vi "RT_Starting_Program.vi"() -> ()   [LabVIEW 2019]
uses:
  <vilib>/Simulation/Scripting/Companion Diagram/SimConfigNode/SimParams.ctl
  <vilib>/Simulation/Scripting/Companion Diagram/SimConfigNode/_simSolvers.ctl
  <vilib>/Simulation/Implementation/Shared/SIMSCR Execution Mode.ctl
  <vilib>/Platform/TimedLoop/XDataNode/timing_clust.ctl
  <vilib>/Platform/TimedLoop/XDataNode/nitl_modes.ctl
  <vilib>/Platform/TimedLoop/XDataNode/wakeup.ctl
  <vilib>/Simulation/Param Hierarchy/Typedefs/SIMPH Param Control Actions.ctl
  <vilib>/Simulation/Scripting/Editor Utilities/SIM subVI tag data.ctl
  <vilib>/Simulation/Scripting/Editor Utilities/SIM subVI execution type.ctl
  <vilib>/Simulation/Implementation/Shared/NILVSim_ParamChanged.vi
  <vilib>/Simulation/Implementation/Shared/NILVSim_FinishedLate.vi
  <vilib>/Simulation/Implementation/Shared/NILVSIM_BeginStep.vi
  <vilib>/Simulation/Utility/Implementation/SIM Halt.vi
  <vilib>/Simulation/Implementation/Shared/SIM Fire Discrete SubVI.vi
  <vilib>/Simulation/SignalDisplay/Implementation/NILVSim Time Waveform.llb/SIM Time Waveform (vector).vi
  <vilib>/Simulation/Implementation/Shared/NILVSim_Manager.vi
  <vilib>/Utility/error.llb/Clear Errors.vi
  <vilib>/Simulation/Implementation/Shared/NILVSim_FinalizeModel.vi
  <vilib>/Simulation/Implementation/Shared/SIM Fire Discrete SubVI (Core).vi
  <vilib>/myRIO/Common/Instrument Driver Framework/myRIO v1.0/UART/vis/myRIO v1.0 Close UART.vi
  <vilib>/FPGAPlugInAG/myRIO-1900/niLvFpga_Open_myRIO-1900.vi
  <vilib>/rvi/interface/common/dynamic/niFpgaDynamicAddResources.vi
  <vilib>/Utility/error.llb/Error Cluster From Error Code.vi
  <vilib>/rvi/errors/niLvFpgaAdjustHostInterfaceError.vi
  <vilib>/Simulation/Implementation/Shared/SIM Unbundle Sim Info.vi
  <vilib>/Simulation/Implementation/Shared/SIMSH Read Queue.vi
  <vilib>/Simulation/Implementation/Shared/NILVSim_Initialize.vi
  SubVIs/Output_Scaling.vi
  SubVIs/Encoder Scaling VI.vi
  <vilib>/Simulation/Utility/Implementation/NILVSim Get Time and IsAcceptedStep.vi
  <vilib>/Simulation/Implementation/Shared/NILVSim_GetModelError.vi
  <vilib>/Simulation/Implementation/Shared/SIM Bundle Sim Info.vi
  <vilib>/FPGAPlugInAG/Dynamic/niLvFpga_Close_Dynamic.vi
  <vilib>/myRIO/Common/Instrument Driver Framework/Utilities/vis/FPGA Ref Manager.vi
  <vilib>/myRIO/Common/Instrument Driver Framework/myRIO v1.0/myRIO v1.0 Reset FPGA.vi
  <vilib>/myRIO/Common/Instrument Driver Framework/myRIO v1.0/IRQ/vis/myRIO v1.0 IRQ Info FGV.vi
  <vilib>/myRIO/Common/Instrument Driver Framework/myRIO v1.0/IRQ/vis/myRIO v1.0 Timer IRQ Info FGV.vi
  <vilib>/myRIO/Common/Instrument Driver Framework/myRIO v1.0/IRQ/vis/myRIO v1.0 ISR Agent.vi
  <vilib>/myRIO/Instrument Drivers/Utilities/vis/Reset Index.vi
  <vilib>/myRIO/Common/Instrument Driver Framework/myRIO v1.0/Resource Manager/vis/myRIO v1.0 Block Write Resource Manager.vi
  <vilib>/rvi/interface/nirviOpenFPGA/nirviOpenFPGA.xnode
  FPGA Bitfiles/SheepdogProject_FPGATarget_FPGAEncoderandPW_gBORoPHN0GY.lvbitx
  <vilib>/rvi/interface/nirviReadWriteControl/nirviReadWriteControl.xnode
  <vilib>/Simulation/Scripting/Companion Diagram/SimConfigNode/SimDog.xnode
  <vilib>/Platform/TimedLoop/XDataNode/XDataNode.xnode
  <vilib>/Simulation/Implementation/XNodeFramework/SimXNode/SimX.xnode
  <vilib>/rvi/interface/nirviCloseFPGA/nirviCloseFPGA.xnode
  <vilib>/rvi/interface/Simulation/niFpgaSimulationCallBeginRW.vi
  <vilib>/myRIO/Instrument Drivers/Utilities/Utilities.lvlib
  NiFpgaLv.dll
  <vilib>/Platform/TimedLoop/XDataNode/XDNodeRunTimeDep.lvlib
  <vilib>/Simulation/Implementation/Shared/NI_SIM_Implementation.lvlib
panel:
  in  "Right Motor Voltage":dbl(slide) scale=-12.0..12.0
  out "Wheel Positions":waveform(dbl)[](graph)=[{"t0"=timestamp(3.854 s since 1904-01-01), "dt"=1.0, "Y"=[0.0]}, {"t0"=timestamp(3.854 s since 1904-01-01), "dt"=1.0, "Y"=[4.309542698753171]}, {"t0"=timestamp(3.854 s since 1904-01-01), "dt"=1.0, "Y"=[2.7199614260015945]}]
  in  "Left Motor Voltage":dbl(slide) scale=-12.0..12.0
  out "Wheel Velocities (inches/sec)":waveform(dbl)[](graph)=[{"t0"=timestamp(3.854 s since 1904-01-01), "dt"=1.0, "Y"=[0.0]}, {"t0"=timestamp(3.854 s since 1904-01-01), "dt"=1.0, "Y"=[4.309542698753171]}, {"t0"=timestamp(3.854 s since 1904-01-01), "dt"=1.0, "Y"=[2.7199614260015945]}]
  in  "Stop":bool
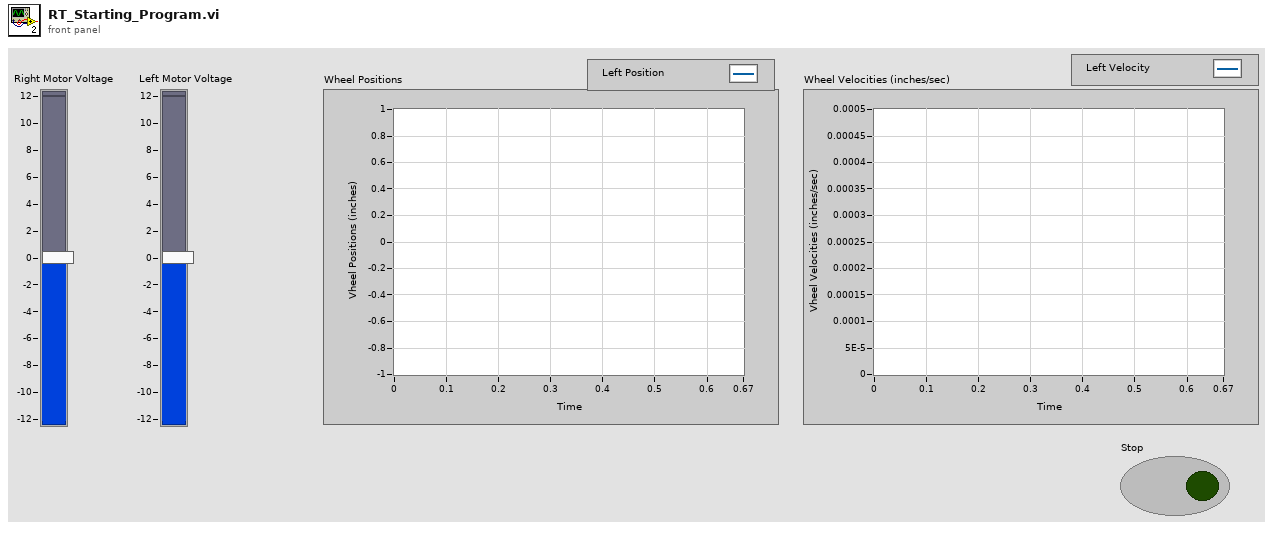
[diagram p1: front panel]
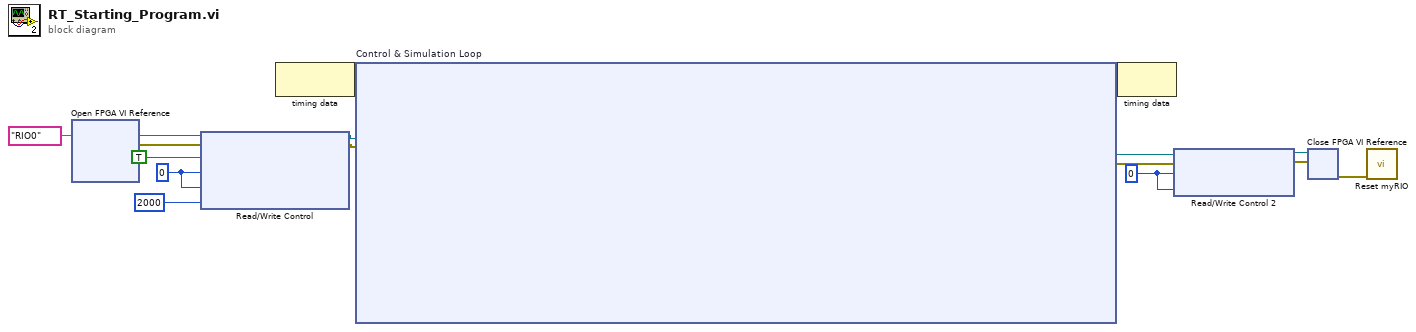
[diagram p0: block diagram]
diagram:
  w10 = i16 0 ("index 2")
  w9 = i16 0 ("Duty Cycle (ticks)")
  n1 = xnode "Open FPGA VI Reference"("resource name"=tag "RIO0") -> ("FPGA VI Reference Out"=w16:refnum<k20>, "error out"=w7:errorcluster)  [unwired: 1 in]
  n2 = xnode "Read/Write Control"("FPGA VI Reference In"=w16, "error in"=w7, "Reset Encoder Position"=TRUE ("Reset Left Encoder Position"), "Motor 1 Duty Cycle"=w10, "Motor 2 Duty Cycle"=w10, "Motor Duty Cycle Period"=i16 2000 ("index 2")) -> ("FPGA VI Reference Out"=w4:refnum<k20>, "error out"=w3:errorcluster)
  n3 = node-c288() -> (w6:variant)  [unwired: 1 in]
  n4 = node-c254 "Control & Simulation Loop"(w6, w4, w3) -> (w5:variant, w2:refnum<k20>, w1:errorcluster)
  n5 = node-c288(w5) -> ()  [unwired: 1 out]
  n6 = xnode ("Read/Write Control 2")("FPGA VI Reference In"=w2, "error in"=w1, "Motor 1 Duty Cycle"=w9, "Motor 2 Duty Cycle"=w9) -> ("FPGA VI Reference Out"=w14:refnum<k20>, "error out"=w12:errorcluster)
  n7 = xnode "Close FPGA VI Reference"("FPGA VI Reference In"=w14, "error in"=w12) -> ("error out"=w13:errorcluster)
  n8 = call <vilib>:"Reset myRIO.vi"("error in (no error)"=w13) -> ()  [unwired: 10 in, 1 out]
